vi "Voice coil response averaging.vi"() -> ()   [LabVIEW 2020]
uses:
  <vilib>/Analysis/baseanly.llb/Mean (DBL).vi
  <vilib>/Analysis/NI_AALBase.lvlib
panel:
  out "mean 2":dbl=0.03825110999999997 format="%0.2f"
  out "transposed array":dbl[][](array[numeric])
  out "Average values over samples 4":dbl[][](graph)
  out "Array 2":dbl[](array[numeric])=[-0.115223, -0.113578, -0.113907, -0.113085, -0.110783, -0.112263, -0.108974, -0.108152, -0.106672, -0.104205, -0.103547, -0.101903, -0.10141, -0.100259, -0.099601, -0.099601, -0.097628, -0.097628, -0.093845, -0.093352, -0.091708, -0.090392, -0.08957, -0.088419, -0.087432, -0.087432, -0.086117, -0.08365, -0.083486, -0.083486, -0.080197, -0.07921, -0.078059, -0.074935, -0.075757, -0.072139, -0.073619, -0.072797, -0.072304, -0.070824, -0.068686, -0.068193, -0.066548, -0.06474, -0.062273, -0.062437, -0.06178, -0.061944, -0.059642, -0.059313, -0.058491, -0.05586, -0.055038, -0.052735, -0.050762, -0.051749, -0.049775, -0.049775, -0.047967, -0.047967, -0.045336, -0.044842, -0.042705, -0.040731, -0.040896, -0.040567, -0.042047, -0.036785, -0.037442, -0.035469, -0.034811, -0.036291, -0.030372, -0.030536, -0.027412, -0.028727, -0.026754, -0.025274, -0.026096, -0.024452, -0.022807, -0.027247, -0.020012, -0.020176, -0.016887, -0.016723, -0.01475, -0.014092, -0.01327, -0.01179, -0.013434, -0.009652, -0.008994, -0.007514, -0.006199, -0.004061, -0.002581, -0.001759, -0.000937, -0.00587, 0.001201, 0.001365, 0.003503, 0.004325, 0.00597, 0.007121, 0.008272, 0.009916, 0.010903, 0.00745, 0.012712, 0.015014, 0.013369, 0.017152, 0.016987, 0.017974, 0.02044, 0.022414, 0.023071, 0.023894, 0.023236, 0.025374, 0.026196, 0.028991, 0.028827, 0.028991, 0.032773, 0.031129, 0.03376, 0.036555, 0.036391, 0.038035, 0.037707, 0.035569, 0.040995, 0.040338, 0.042475, 0.044449, 0.044777, 0.048066, 0.047737, 0.049711, 0.051684, 0.050533, 0.052342, 0.052342, 0.053986, 0.056453, 0.057933, 0.059248, 0.060235, 0.060564, 0.062701, 0.062866, 0.064675, 0.06451, 0.066812, 0.066319, 0.06895, 0.070595, 0.070923, 0.072897, 0.073883, 0.074541, 0.075528, 0.074706, 0.079474, 0.078323, 0.079474, 0.081941, 0.081612, 0.08523, 0.084243, 0.086545, 0.086052, 0.08819, 0.085394, 0.090163, 0.091807, 0.092465, 0.094109, 0.096083, 0.09674, 0.099372, 0.099865, 0.103647, 0.101838, 0.101838, 0.103811, 0.103976, 0.105127, 0.107758, 0.108251, 0.110553, 0.11302, 0.112033, 0.113678, 0.113842, 0.115322, 0.117295, 0.115487, 0.119762, 0.119598, 0.124366, 0.123215, 0.124366, 0.12486, 0.125517, 0.12782, 0.129464, 0.128971, 0.130944, 0.133904, 0.132588, 0.136371, 0.135877, 0.136864, 0.136864, 0.138344, 0.13933, 0.14081, 0.142619, 0.143277, 0.144099, 0.146237, 0.147059, 0.149361, 0.150348, 0.150512, 0.149526, 0.152157, 0.152979, 0.154952, 0.154788, 0.156925, 0.159885, 0.16005, 0.161694, 0.162845, 0.159885, 0.165147, 0.164983, 0.165805, 0.167943, 0.168601, 0.169423, 0.171396, 0.173863, 0.172054, 0.175014, 0.177152, 0.178303, 0.177809, 0.180934, 0.181591, 0.181591, 0.184058, 0.178303, 0.185867, 0.187511, 0.186525, 0.18932, 0.189649, 0.190965, 0.192445, 0.191951, 0.194582, 0.19524, 0.197542, 0.199351, 0.198858, 0.201818, 0.20116, 0.203791, 0.205106, 0.204778, 0.204778, 0.20708, 0.209875, 0.21004, 0.211191, 0.213164, 0.212671, 0.214973, 0.216453, 0.217768, 0.217439, 0.21859, 0.219577, 0.222701, 0.222701, 0.224839, 0.224181, 0.225497, 0.22599, 0.228128, 0.228457, 0.23487, 0.232568, 0.23339, 0.230759, 0.23635, 0.236679, 0.238488, 0.23931, 0.240461, 0.245394, 0.241941, 0.24375, 0.24523, 0.245559, 0.248519, 0.250821, 0.249176, 0.250821, 0.25115, 0.253123, 0.254109, 0.255918, 0.257234, 0.259536, 0.26118, 0.260358, 0.261674, 0.263154, 0.263647, 0.265456, 0.264798, 0.267594, 0.269238, 0.267429, 0.271211, 0.272033, 0.27302, 0.2745, 0.27598, 0.27746, 0.27746, 0.280913, 0.280255, 0.280749, 0.28338, 0.283215, 0.284531, 0.286175, 0.286175, 0.288313, 0.289464, 0.292095, 0.291602, 0.293411, 0.293411, 0.296371, 0.296371, 0.297686, 0.29933, 0.30081, 0.29785, 0.301961, 0.30377, 0.304921, 0.305908, 0.30673, 0.308046, 0.310183, 0.311335, 0.311828, 0.313637, 0.313801, 0.315939, 0.316103, 0.317583, 0.319392, 0.319721, 0.321694, 0.322516, 0.319228, 0.324819, 0.32597, 0.326956, 0.328107, 0.329587, 0.330081, 0.332054, 0.330903, 0.333205, 0.335507, 0.335014, 0.337645, 0.338303, 0.33896, 0.341263, 0.341263, 0.344387, 0.345045, 0.345867, 0.347676, 0.34784, 0.350471, 0.349813, 0.351293, 0.352773, 0.353431, 0.348498, 0.356227, 0.357871, 0.359515, 0.36116, 0.360667, 0.367573, 0.362311, 0.364942, 0.369217, 0.367244, 0.366586, 0.367902, 0.371026, 0.370368, 0.372342, 0.374479, 0.374808, 0.376288, 0.377933, 0.37859, 0.380728, 0.380235, 0.381221, 0.385661, 0.384181, 0.385497, 0.386812, 0.387635, 0.388621, 0.39043, 0.391252, 0.393226, 0.39191, 0.393719, 0.395528, 0.396186, 0.398159, 0.400297, 0.406216, 0.401119, 0.402928, 0.397501, 0.405065, 0.405887, 0.407532, 0.408683, 0.410492, 0.41115, 0.411972, 0.412136, 0.409998, 0.415261, 0.418056, 0.417892, 0.418878, 0.420687, 0.421345, 0.423811, 0.423811, 0.419372, 0.426278, 0.426607, 0.429073, 0.430225, 0.431211, 0.431869, 0.432527, 0.434829, 0.432362, 0.435816, 0.437295, 0.439762, 0.439762, 0.441735, 0.441571, 0.443051, 0.444531, 0.439104, 0.448149, 0.448313, 0.448806, 0.450944, 0.451273, 0.452917, 0.453411, 0.455713, 0.456042, 0.456699, 0.459166, 0.46081, 0.46081, 0.463606, 0.464428, 0.46377, 0.466072, 0.466895, 0.467388, 0.470019, 0.469526, 0.472157, 0.473472, 0.476103, 0.475446, 0.476432, 0.477419, 0.479228, 0.479557, 0.481365, 0.482188, 0.48005, 0.483996, 0.486134, 0.487121, 0.488436, 0.488601, 0.49041, 0.491725, 0.493041, 0.494192, 0.490574, 0.496494, 0.497645, 0.499125, 0.500276, 0.500769, 0.500276, 0.503894, 0.504058, 0.510471, 0.507018, 0.50784, 0.510307, 0.509978, 0.512444, 0.512938, 0.512938, 0.514747, 0.511458, 0.517707, 0.518529, 0.519844, 0.520173, 0.522311, 0.526093, 0.523955, 0.524777, 0.526751, 0.528066, 0.527737, 0.53004, 0.531848, 0.532999, 0.528231, 0.534973, 0.533328, 0.537768, 0.53859, 0.538755, 0.540564, 0.541715, 0.543359, 0.539906, 0.545004, 0.547306, 0.548128, 0.549279, 0.549937, 0.550759, 0.552239, 0.552897, 0.55487, 0.555363, 0.556679, 0.558323, 0.559145, 0.561119, 0.560296, 0.561941, 0.564407, 0.56079, 0.565723, 0.567696, 0.56819, 0.569176, 0.571478, 0.578714, 0.572958, 0.575096, 0.576905, 0.577069, 0.578714, 0.579207, 0.580523, 0.581509, 0.582167, 0.58414, 0.586278, 0.586771, 0.586936, 0.586936, 0.586607, 0.590389, 0.593349, 0.592691, 0.593184, 0.595651, 0.596638, 0.597624, 0.599762, 0.600255, 0.601078, 0.602886, 0.603051, 0.604366, 0.605846, 0.605189, 0.608148, 0.609957, 0.609793, 0.612424, 0.613575, 0.614726, 0.615877, 0.613904, 0.613246, 0.619659, 0.618179, 0.496329, 0.13785, -0.270125, -0.479293, -0.526651, -0.539313, -0.540958, -0.543424, -0.54326, -0.540629, -0.53882, -0.534709, -0.529447, -0.527145, -0.529118, -0.528789, -0.527638, -0.533393, -0.5329, -0.532242, -0.530269, -0.526158, -0.520896, -0.516785, -0.515798, -0.514812, -0.516785, -0.519087, -0.520074, -0.520403, -0.520403, -0.516456, -0.51251, -0.508234, -0.504288, -0.504288, -0.503137, -0.504123, -0.510207, -0.50807, -0.507248, -0.506754, -0.502314, -0.500012, -0.501163, -0.489817, -0.49179, -0.492941, -0.492777, -0.492941, -0.495901, -0.495243, -0.491626, -0.489652, -0.485541, -0.483239, -0.479786, -0.477319, -0.478306, -0.480937, -0.484884, -0.482088, -0.481595, -0.478471, -0.484061, -0.473044, -0.468933, -0.46696, -0.466302, -0.467289, -0.468111, -0.468604, -0.469755, -0.467289, -0.46548, -0.462849, -0.456107, -0.456271, -0.453969, -0.452818, -0.457587, -0.455778, -0.456271, -0.4566, -0.453147, -0.451502, -0.445089, -0.44476, -0.441636, -0.439992, -0.441143, -0.440978, -0.442129, -0.443774, -0.4418, -0.441143, -0.439005, -0.433907, -0.431934, -0.43029, -0.428316, -0.428974, -0.429632, -0.429467, -0.431112, -0.430947, -0.427659, -0.423712, -0.422561, -0.418614, -0.41697, -0.416148, -0.415819, -0.416312, -0.417134, -0.416312, -0.415819, -0.414503, -0.410392, -0.409241, -0.404966, -0.404801, -0.403321, -0.402828, -0.404637, -0.404144, -0.404144, -0.401841, -0.40069, -0.400033, -0.395593, -0.391482, -0.391811, -0.390002, -0.390824, -0.391646, -0.390988, -0.391482, -0.390495, -0.38622, -0.383589, -0.385891, -0.379478, -0.378327, -0.376682, -0.377504, -0.379642, -0.379807, -0.377833, -0.376682, -0.374709, -0.370598, -0.369118, -0.365665, -0.365336, -0.365336, -0.364678, -0.359087, -0.365665, -0.364185, -0.36402, -0.358923, -0.356949, -0.355798, -0.353496, -0.352838, -0.355469, -0.353661, -0.352838, -0.351194, -0.352016, -0.349221, -0.34659, -0.344945, -0.34215, -0.340505, -0.339519, -0.339354, -0.340176, -0.342643, -0.339848, -0.338697, -0.335737, -0.332777, -0.332941, -0.328501, -0.328008, -0.327186, -0.323732, -0.327843, -0.326528, -0.326199, -0.325706, -0.322253, -0.320773, -0.318799, -0.314031, -0.313866, -0.315017, -0.314359, -0.315346, -0.313702, -0.313373, -0.313373, -0.310084, -0.306466, -0.30548, -0.304, -0.300711, -0.303013, -0.302026, -0.300875, -0.302355, -0.300711, -0.298902, -0.297751, -0.294791, -0.291009, -0.289365, -0.289529, -0.289365, -0.287391, -0.292324, -0.288871, -0.286569, -0.286076, -0.282787, -0.280649, -0.279663, -0.278018, -0.276045, -0.283609, -0.276867, -0.27588, -0.275716, -0.274072, -0.271605, -0.270783, -0.267987, -0.265192, -0.269138, -0.264041, -0.262725, -0.263876, -0.263054, -0.262232, -0.262232, -0.259436, -0.257134, -0.253517, -0.253188, -0.253845, -0.255819, -0.250392, -0.250886, -0.250063, -0.248419, -0.24661, -0.247268, -0.243486, -0.242006, -0.240033, -0.247103, -0.239539, -0.239704, -0.239539, -0.237895, -0.235757, -0.235264, -0.231975, -0.229673, -0.229837, -0.228193, -0.226548, -0.225397, -0.22622, -0.227042, -0.225726, -0.22326, -0.222766, -0.220793, -0.21734, -0.216353, -0.217011, -0.213558, -0.213887, -0.213722, -0.213393, -0.212735, -0.210269, -0.209282, -0.20698, -0.202211, -0.203198, -0.201718, -0.200402, -0.204185, -0.200567, -0.20106, -0.199745, -0.195469, -0.196949, -0.193496, -0.191852, -0.189714, -0.190207, -0.188069, -0.189221, -0.188069, -0.185932, -0.183958, -0.18511, -0.182314, -0.180341, -0.182807, -0.177216, -0.177545, -0.176559, -0.174914, -0.175243, -0.172941, -0.172777, -0.170474, -0.168666, -0.167514, -0.166199, -0.165377, -0.163732, -0.162252, -0.163568, -0.162581, -0.163075, -0.15995, -0.157813, -0.156497, -0.154853, -0.153044, -0.152715, -0.150906, -0.150413, -0.150413, -0.147124, -0.148439, -0.147617, -0.146466, -0.143342, -0.141204, -0.140217, -0.138902, -0.136271, -0.138902, -0.137093, -0.136271, -0.136271, -0.132818, -0.132818, -0.130844, -0.129036, -0.127884, -0.126569, -0.126404, -0.125911, -0.125418, -0.128707, -0.122458, -0.121471, -0.120156, -0.117689, -0.116045]
  in  "Number of Samples to average over":i32=10
  out "Average values over samples 2":dynamicdata(graph)=[{"t0"=timestamp(0 s since 1904-01-01), "dt"=1.0, "Y"=array[1000 elements], "attributes"=variant("NI_ChannelName"=variant(string "Untitled"), "NI_ExpIsRelativeTime"=variant(bool TRUE), "NI_ExpStartTimeStamp"=variant(timestamp timestamp(3780666649.7478743 s since 1904-01-01)), "NI_ExpTimeStamp"=variant(timestamp timestamp(0 s since 1904-01-01)), "NI_ExpXDimension"=variant(string "t"), "NI_UnitDescription"=variant(string "V"))}]
  out "Average values over samples":dbl[](graph)=[0.0, 0.0, 0.0, 0.0, 0.0, 0.0, 0.0, 0.0, 0.0, 0.03825110999999997]
  out "path":path=path "C:/Users/htm22/Documents/LabVIEW Data/voicecoil_010.lvm"
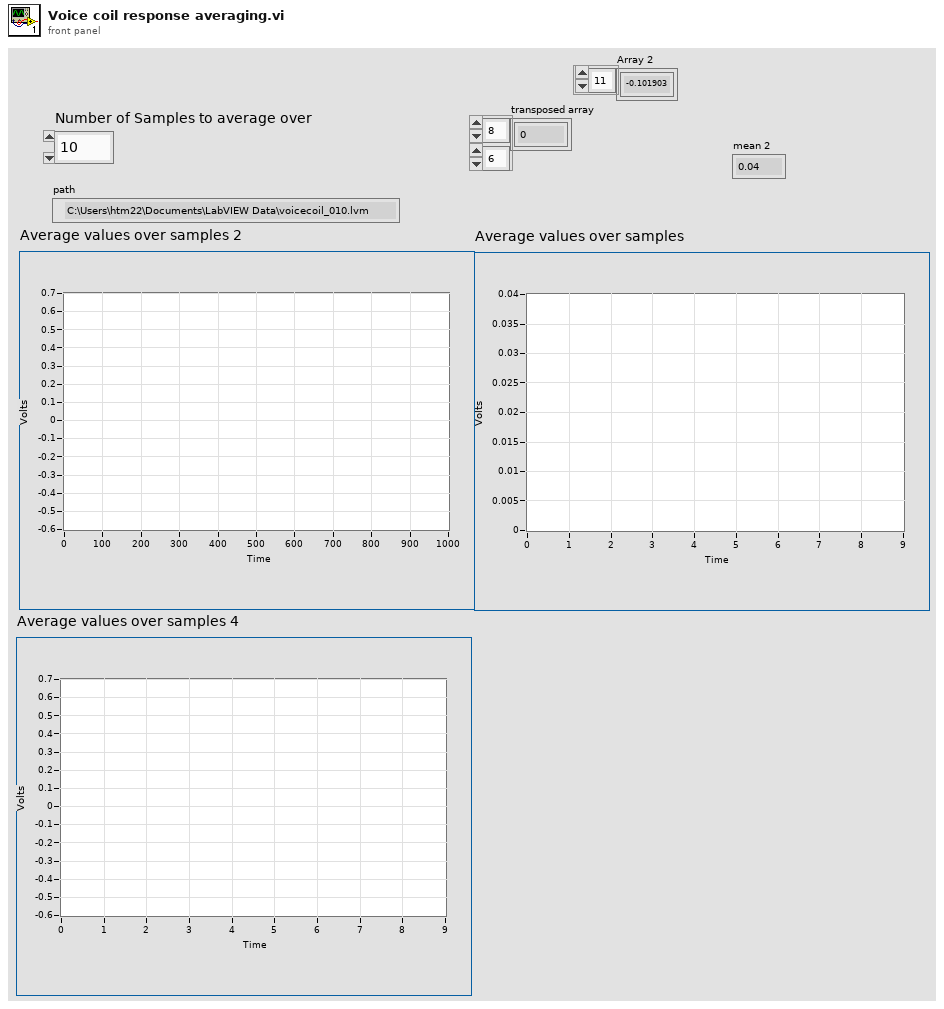
[diagram p1: front panel]
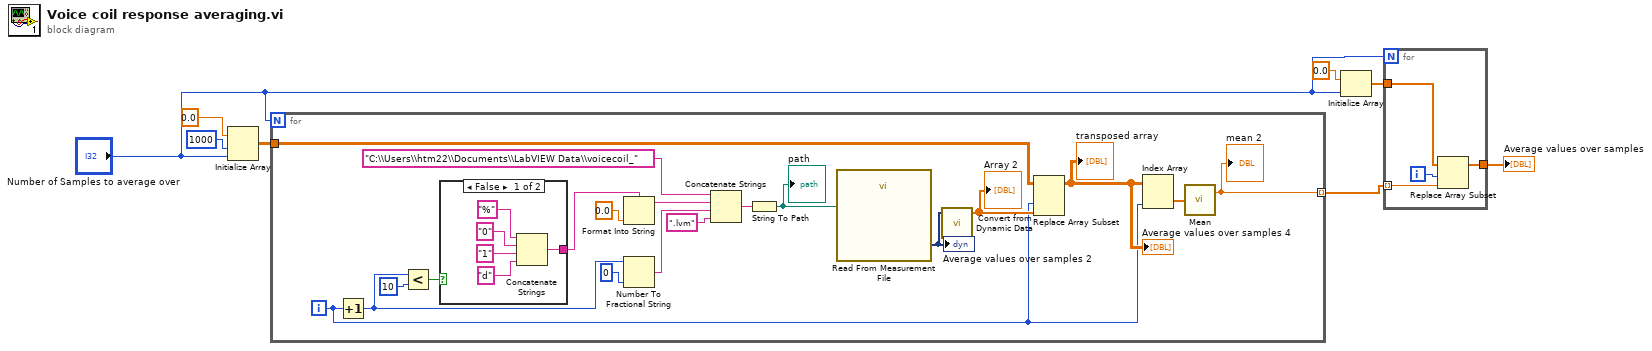
[diagram p0: block diagram]
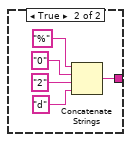
[diagram p2: hidden frame]
diagram:
  n1 = Initialize Array(0.0 ("element"), 1000 ("dimension size"), "Number of Samples to average over") -> (w4:dbl[][])
  n2 = for {
    N: "Number of Samples to average over" -> [_]
    tunnel: w4 -> [w13]
    tunnel: [w11] -> w3 mode=indexing
    i -> [w9]
    n3 = Increment(x=w9) -> (x+1=w19:i32)
    n4 = Less?(x=w19, y=10) -> (x < y?=w17:bool)
    n5 = case shown="False" w17 {
      tunnel: [w28 w33] -> w16
      frame False {
        n6 = Concatenate Strings("%" ("string"), "0" ("string"), "1" ("string"), "d" ("string")) -> (w28:string)
      }
      frame True {
        n7 = Concatenate Strings("%" ("string"), "0" ("string"), "2" ("string"), "d" ("string")) -> (w33:string)
      }
    }
    n8 = Format Into String(format string=w16, 0.0 ("input 1")) -> (resulting string=w20:string)  [unwired: 2 in, 1 out]
    n9 = Number To Fractional String(number=w19, precision (6)=i16 0) -> (F-format string=w21:string)  [unwired: 2 in]
    n10 = Concatenate Strings("C:\\Users\\htm22\\Documents\\LabVIEW Data\\voicecoil_" ("string"), w20, w21, ".lvm") -> (w26:string)
    n11 = String To Path(string=w26) -> (path=w27:path)
    "path" <- w27
    n12 = call "Read From Measurement File"("Filename"=w27) -> ("Signals"=w15:dynamicdata)  [unwired: 5 in, 5 out]
    "Average values over samples 2" <- w15
    n13 = call "Convert from Dynamic Data"("Dynamic Data Type"=w15) -> ("Array"=w14:dbl[])  [unwired: 3 in]
    "Array 2" <- w14
    n14 = Replace Array Subset(array=w13, new element=w14, index (col)=w9) -> (w10:dbl[][])  [unwired: 1 in]
    "Average values over samples 4" <- w10
    "transposed array" <- w10
    n15 = Index Array(array=w10, index (col)=w9) -> (element=w12:dbl[])  [unwired: 1 in]
    n16 = call-poly <vilib>:"Mean.vi"("X"=w12) -> ("mean"=w11:dbl)  [unwired: 1 out]
    "mean 2" <- w11
  }
  n17 = Initialize Array(0.0 ("element"), "Number of Samples to average over") -> (w6:dbl[])
  n18 = for {
    N: "Number of Samples to average over" -> [_]
    tunnel: [w41] -> w5
    tunnel: w3 -> [w38] mode=indexing
    tunnel: w6 -> [w39]
    i -> [w40]
    n19 = Replace Array Subset(array=w39, new element=w38, index=w40) -> (w41:dbl[])
  }
  "Average values over samples" <- w5
